vi "Init UDP Communication.vi"(8 "error in (no error)":errorcluster, 10 "RT State Variables In":T1 {"Settings"."Tx Packet Info"."Endianness" items=["big-endian"=0, "little-indian"=2]; "Settings"."Rx Packet Info"."Endianness" items=["big-endian"=0, "little-indian"=2]}) -> (0 "error out":errorcluster, 2 "RT State Variables Out":T1 {"Settings"."Tx Packet Info"."Endianness" items=["big-endian"=0, "little-indian"=2]; "Settings"."Rx Packet Info"."Endianness" items=["big-endian"=0, "little-indian"=2]})   [LabVIEW 2016, in "UDP-Custom-Device Engine.lvlib"]
uses:
  UDP-Custom-Device Engine.lvlib
  Shared/Compiled.Settings.ctl
  Shared/UDP-Custom-Device Shared.lvlib
  <vilib>/NI/NIVS Inline Async API/_VS Inline Async API/VS Inline Async API/VS Inline Async API.lvclass
  <vilib>/NI/NIVS Inline Async API/_Data Access Engine/Access Type Classes/Write/Write.lvclass
  <vilib>/NI/NIVS Inline Async API/_Data Access Engine/Data Access Engine/Types/Write.DVR.ctl
  <vilib>/NI/NIVS Inline Async API/_Data Access Engine/Data Access Engine/Data Access Engine.lvclass
  <vilib>/NI/NIVS Inline Async API/_Data Access Engine/Access Type Classes/Read/Read.lvclass
  <vilib>/NI/NIVS Inline Async API/_Data Access Engine/Data Access Engine/Types/Read.DVR.ctl
  RTStateVariables.ctl
  Shared/Rx.PacketInfo.ctl
  Shared/Tx.PacketInfo.ctl
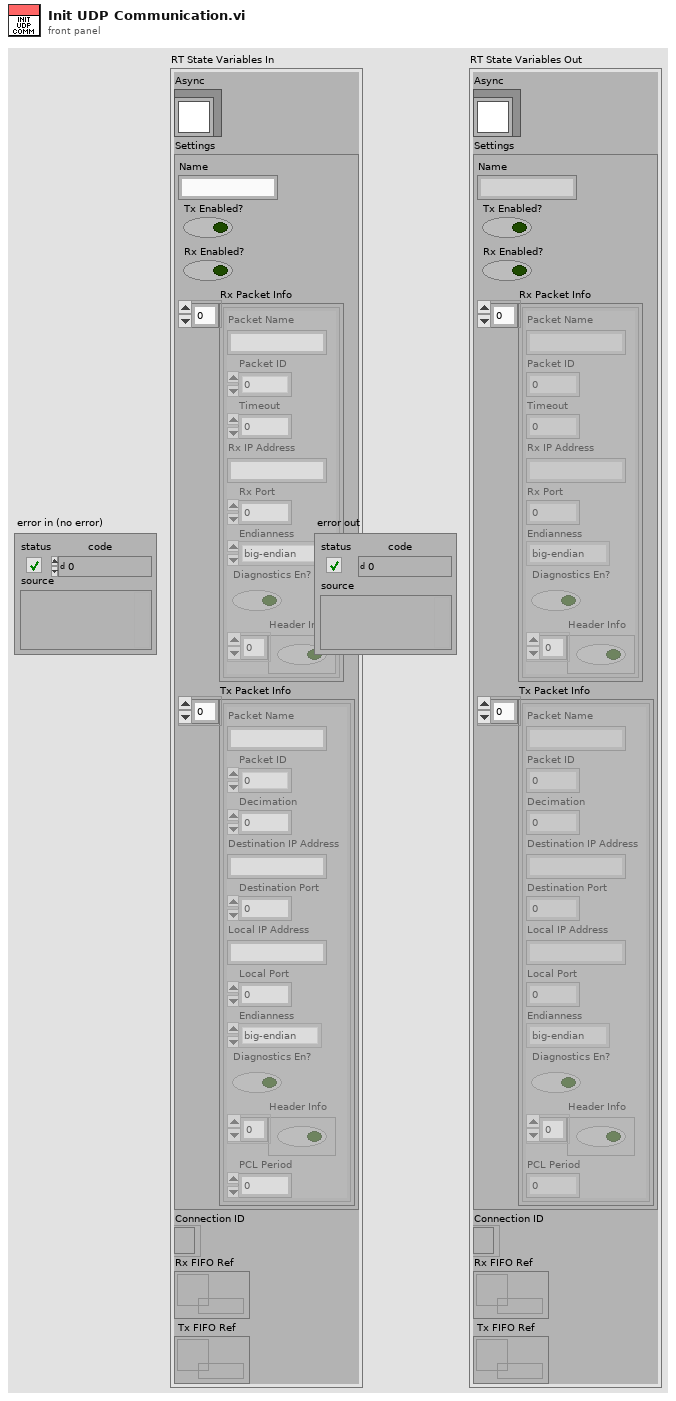
[diagram p1: front panel]
types:
  T1 = typedef "UDP-Custom-Device Engine.lvlib/RTStateVariables.ctl" = cluster{"Async":refnum<class "VS Inline Async API.lvclass">, "Settings":T2, "Connection ID":refnum<k16>, "Rx FIFO Ref":T5, "Tx FIFO Ref":T6}
  T2 = typedef "UDP-Custom-Device Shared.lvlib/Compiled.Settings.ctl" = cluster{"Name":string, "Tx Enabled?":bool, "Rx Enabled?":bool, "Rx Packet Info":T3[], "Tx Packet Info":T4[]}
  T3 = typedef "UDP-Custom-Device Shared.lvlib/Rx.PacketInfo.ctl" = cluster{"Packet Name":string, "Packet ID":i32, "Timeout":i32, "Rx IP Address":string, "Rx Port":i32, "Endianness":u16, "Diagnostics En?":bool, "Header Info":bool[]}
  T4 = typedef "UDP-Custom-Device Shared.lvlib/Tx.PacketInfo.ctl" = cluster{"Packet Name":string, "Packet ID":i32, "Decimation":i32, "Destination IP Address":string, "Destination Port":i32, "Local IP Address":string, "Local Port":i32, "Endianness":u16, "Diagnostics En?":bool, "Header Info":bool[], "PCL Period":u32}
  T5 = typedef "Data Access Engine.lvlib/Data Access Engine.lvclass/Write.DVR.ctl" = refnum<data-value>
  T6 = typedef "Data Access Engine.lvlib/Data Access Engine.lvclass/Read.DVR.ctl" = refnum<data-value>
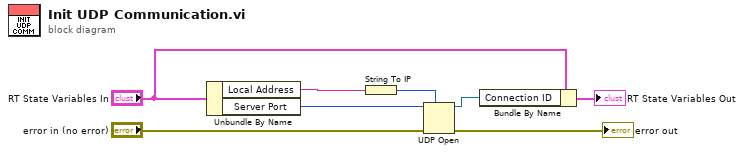
[diagram p0: block diagram]
diagram:
  n1 = Unbundle By Name("RT State Variables In") -> ("Local Address"=w6:string, "Server Port"=w3:u16)
  n2 = String To IP(1:w6) -> (0:w5:u32)
  n3 = UDP Open(7:w5, 8:"error in (no error)", 11:w3) -> (port=w4:refnum<k16>, 0:→"error out":errorcluster)  [unwired: 2 in, 1 out]
  n4 = Bundle By Name(cluster="RT State Variables In", "Connection ID"=w4) -> (→"RT State Variables Out":T1)
